vi ".INI READ.vi"(11 "KEY":string) -> (0 "COM":string, 1 "MODE":string, 2 "TEST MODE":string, 3 "OUT":dbl, 4 "TIME":dbl, 6 "AUTH KEY":string, 8 "error out":errorcluster, 10 "Serail No":cluster{"Serial Number":T1})   [LabVIEW 2021]
uses:
  SERIAL N0.ctl
  <vilib>/Utility/config.llb/Read Key (Double).vi
  <vilib>/Utility/config.llb/Read Key (String).vi
  <vilib>/Utility/config.llb/NI_LVConfig.lvlib
panel:
  in  "Serial No 2":cluster{"Serial Number":T1}
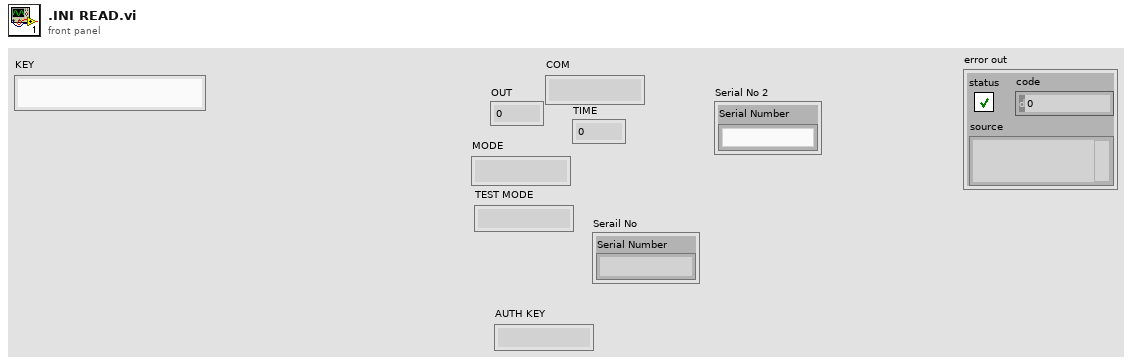
[diagram p1: front panel]
types:
  T1 = typedef "SERIAL N0.ctl" = string
  T2 = typedef "NI_LVConfig.lvlib/Config Data RefNum.ctl" = refnum<k1>
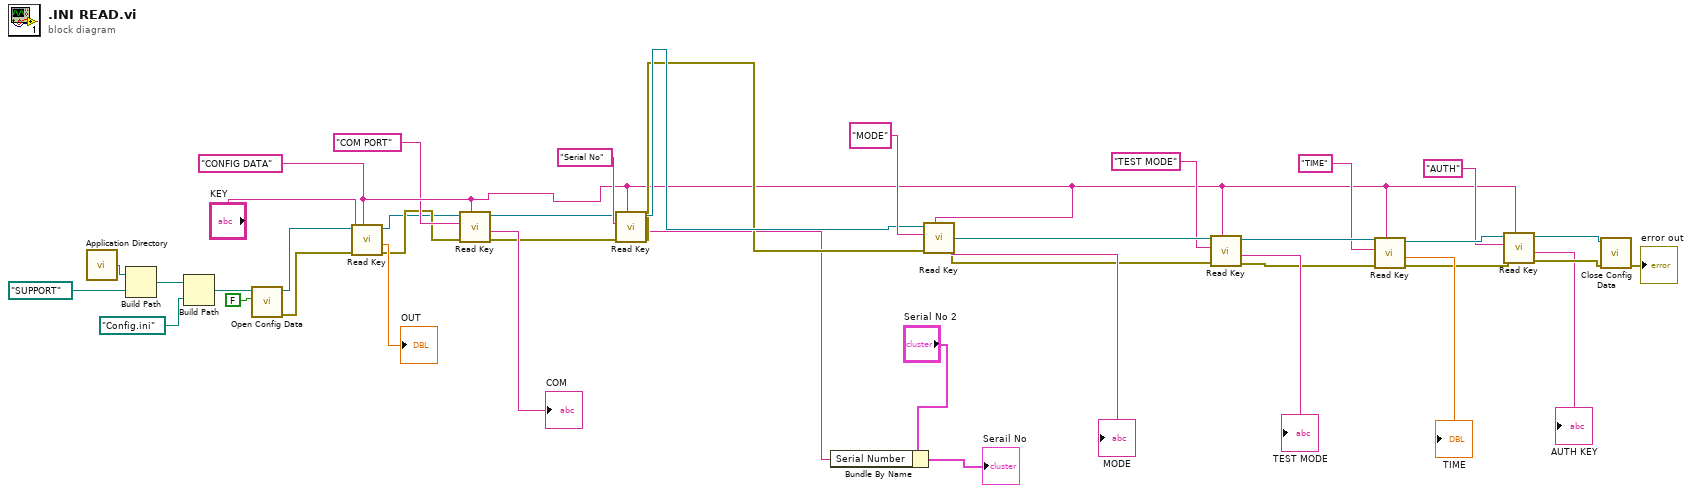
[diagram p0: block diagram]
diagram:
  w7 = "CONFIG DATA" ("section")
  n1 = call <vilib>:"Application Directory.vi"() -> ("Application Directory"=w39:path)
  n2 = Build Path(base path=w39, name or relative path=path "SUPPORT") -> (appended path=w40:path)
  n3 = Build Path(base path=w40, name or relative path=path "Config.ini") -> (appended path=w34:path)
  n4 = call <vilib>:"Open Config Data.vi"("create file if necessary (T)"=FALSE, "configuration file path"=w34) -> ("error out"=w35:errorcluster, "refnum"=w36:T2)  [unwired: 7 in, 1 out]
  n5 = call-poly <vilib>:"Read Key.vi"("section"=w7, "error in (no error)"=w35, "key"="KEY", "refnum"=w36) -> ("error out"=w4:errorcluster, "value"=→"OUT":dbl, "refnum out"=w2:T2)  [unwired: 4 in, 1 out]
  n6 = call-poly <vilib>:"Read Key.vi"("section"=w7, "error in (no error)"=w4, "key"="COM PORT", "refnum"=w2) -> ("error out"=w3:errorcluster, "value"=→"COM":string, "refnum out"=w1:T2)  [unwired: 4 in, 1 out]
  n7 = call-poly <vilib>:"Read Key.vi"("section"=w7, "error in (no error)"=w3, "key"="Serial No", "refnum"=w1) -> ("error out"=w9:errorcluster, "value"=w8:string, "refnum out"=w11:T2)  [unwired: 4 in, 1 out]
  n8 = Bundle By Name(cluster="Serial No 2", "Serial Number"=w8) -> (→"Serail No":cluster{"Serial Number":T1})
  n9 = call-poly <vilib>:"Read Key.vi"("section"=w7, "error in (no error)"=w9, "key"="MODE", "refnum"=w11) -> ("error out"=w27:errorcluster, "value"=→"MODE":string, "refnum out"=w28:T2)  [unwired: 4 in, 1 out]
  n10 = call-poly <vilib>:"Read Key.vi"("section"=w7, "error in (no error)"=w27, "key"="TEST MODE", "refnum"=w28) -> ("error out"=w23:errorcluster, "value"=→"TEST MODE":string, "refnum out"=w24:T2)  [unwired: 4 in, 1 out]
  n11 = call-poly <vilib>:"Read Key.vi"("section"=w7, "error in (no error)"=w23, "key"="TIME", "refnum"=w24) -> ("error out"=w19:errorcluster, "value"=→"TIME":dbl, "refnum out"=w20:T2)  [unwired: 4 in, 1 out]
  n12 = call-poly <vilib>:"Read Key.vi"("section"=w7, "error in (no error)"=w19, "key"="AUTH", "refnum"=w20) -> ("error out"=w18:errorcluster, "value"=→"AUTH KEY":string, "refnum out"=w17:T2)  [unwired: 4 in, 1 out]
  n13 = call <vilib>:"Close Config Data.vi"("error in (no error)"=w18, "refnum"=w17) -> ("error out"=→"error out":errorcluster)  [unwired: 8 in, 1 out]
